vi "Disable UI.vi"(8 "error in (no error)":errorcluster, 11 "Operator UI Actor in":refnum<class "Client UI.lvclass">) -> (0 "error out":errorcluster, 3 "Operator UI Actor out":refnum<class "Client UI.lvclass">)   [LabVIEW 2026, in "Client UI.lvlib" / "Client UI.lvclass"]
uses:
  Client UI.lvclass
  Client UI.lvclass/Client UI.ctl
  MAL-Framework/user.lib/Common Components/Msmt UI/Measurement UI.lvclass
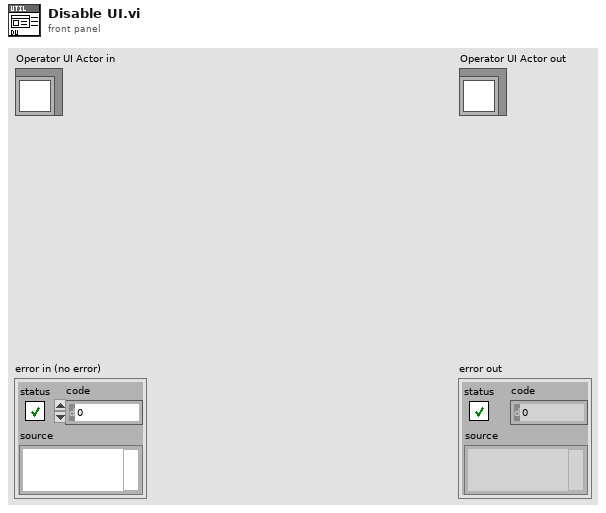
[diagram p1: front panel]
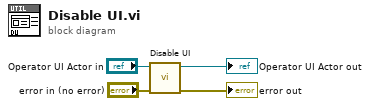
[diagram p0: block diagram]
diagram:
  n1 = call-parent "Disable UI.vi"("error in (no error)"="error in (no error)", "Operator UI Actor in"="Operator UI Actor in") -> ("error out"=→"error out":errorcluster, "Operator UI Actor out"=→"Operator UI Actor out":refnum<class "Client UI.lvclass">)  [unwired: 8 in]
